vi "3-2-1 LabVIEW WebSocket TX.vi"() -> ()   [LabVIEW 2020]
uses:
  state.ctl
  <vilib>/addons/WebSockets-API-master/WebSockets/WebSocket Client/WebSocket Client.lvclass
  C:/Program Files (x86)/National Instruments/LabVIEW 2020/vi.lib/addons/WebSockets-API-master/WebSockets/WebSocket/WebSocket.lvclass
  <vilib>/addons/WebSockets-API-master/WebSockets/WebSocket/WebSocket.lvclass
panel:
  in  "Stop":bool
  out "connection error?":bool
  out "sensor_data":T1={"temperature"=60.0, "pressure"=1.2, "motor"=FALSE, "status"="RUNNING", "timestamp"="21:38:10"}
  out "connect?":bool
  in  "WebSockets URL":string="ws://localhost:8000/ws/labview"
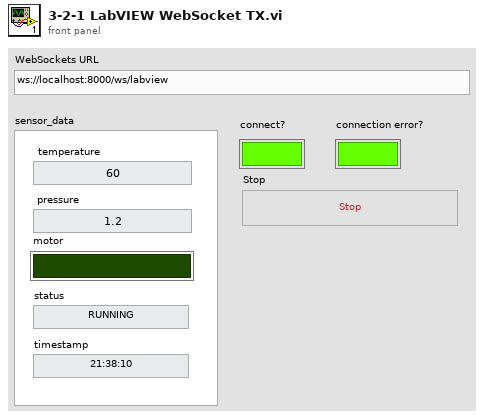
[diagram p1: front panel]
types:
  T1 = cluster{"temperature":dbl, "pressure":dbl, "motor":bool, "status":string, "timestamp":string}
  T2 = typedef "state.ctl" = enum16{"CONNECT", "WRITE_DATA", "READ_DATA", "DISCONNECT"}
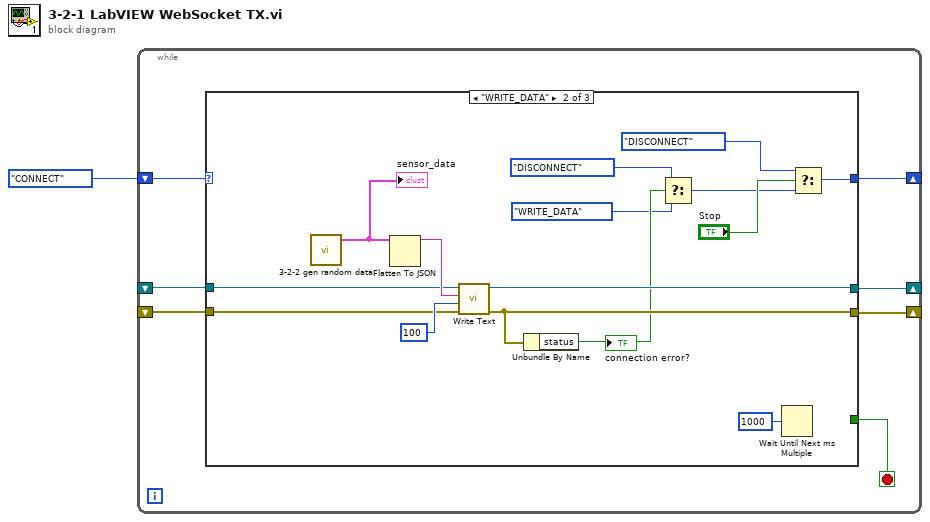
[diagram p0: block diagram]
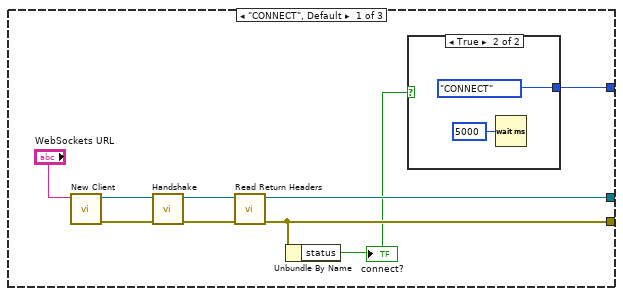
[diagram p2: hidden frame]
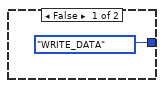
[diagram p3: hidden frame]
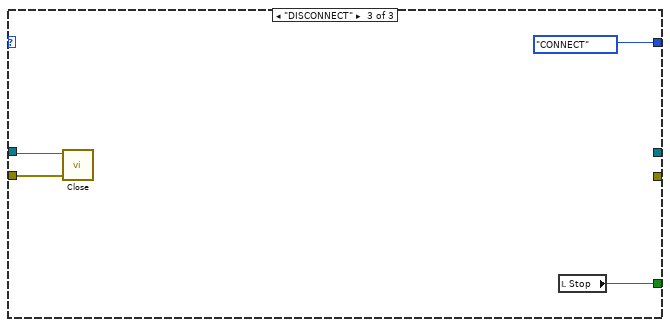
[diagram p4: hidden frame]
diagram:
  n1 = while {
    shift-right: [w5] -> _
    shift-left: state."CONNECT" -> [w8]
    shift-right: [w7] -> _
    shift-left: _ -> [w4]
    shift-right: [w6] -> _
    shift-left: _ -> [w3]
    stop <- w2 stop-if-true
    n2 = case shown="\"WRITE_DATA\"" w8 {
      tunnel: [w12 w31 _] -> w7
      tunnel: [w11 w30 _] -> w6
      tunnel: [w9 w22 state."CONNECT"] -> w5
      tunnel: w4 -> [_ w33 w39]
      tunnel: w3 -> [_ w32 w38]
      tunnel: [_ _ w37] -> w2
      frame "CONNECT", Default {
        n3 = call <vilib>:"New Client.vi"("WebSocket URL"="WebSockets URL") -> ("error out"=w13:errorcluster, "WebSocket Client out"=w15:refnum<class "WebSocket Client.lvclass">)  [unwired: 9 in]
        n4 = call-dynamic "Handshake.vi"("error in (no error)"=w13, "WebSocket Client in"=w15) -> ("error out"=w16:errorcluster, "WebSocket Client out"=w17:refnum<class "WebSocket Client.lvclass">)  [unwired: 8 in]
        n5 = call <vilib>:"Read Return Headers.vi"("error in (no error)"=w16, "WebSocket in"=w17) -> ("error out"=w11:errorcluster, "WebSocket out"=w12:refnum<class "WebSocket Client.lvclass">)  [unwired: 7 in, 1 out]
        n6 = Unbundle By Name(w11) -> ("status"=w10:bool)
        "connect?" <- w10
        n7 = case shown="True" w10 {
          tunnel: [state."WRITE_DATA" state."CONNECT"] -> w9
          frame False {
          }
          frame True {
            n8 = Wait (ms)(milliseconds to wait=u32 5000) -> ()  [unwired: 1 out]
          }
        }
      }
      frame "WRITE_DATA" {
        n9 = call "3-2-2 gen random data.vi"() -> ("output cluster"=w21:T1)  [unwired: 11 in]
        "sensor_data" <- w21
        n10 = Flatten To JSON(anything=w21) -> (JSON string=w35:string)  [unwired: 2 in, 1 out]
        n11 = call-dynamic "Write Text.vi"("error in (no error)"=w32, "timeout ms (5000)"=100, "String Data"=w35, "WebSocket in"=w33) -> ("error out"=w30:errorcluster, "WebSocket out"=w31:refnum<class "WebSocket Client.lvclass">)  [unwired: 6 in]
        n12 = Unbundle By Name(w30) -> ("status"=w28:bool)
        "connection error?" <- w28
        n13 = Select(t=state."DISCONNECT", s=w28, f=state."WRITE_DATA") -> (s? t:f=w24:T2)
        n14 = Wait Until Next ms Multiple(millisecond multiple=u32 1000) -> ()  [unwired: 1 out]
        n15 = Select(t=state."DISCONNECT", s="Stop", f=w24) -> (s? t:f=w22:T2)
      }
      frame "DISCONNECT" {
        n16 = call-dynamic "Close.vi"("error in (no error)"=w38, "WebSocket in"=w39) -> ()  [unwired: 9 in, 1 out]
        n17 = local read "Stop"() -> (w37:bool)
      }
    }
  }
